vi "GV-SetSamplesDots.vi"(8 "error in (no error)":errorcluster, 11 "Gviewer in":refnum<class "Gviewer.lvclass">) -> (0 "error out":errorcluster, 3 "Gviewer out":refnum<class "Gviewer.lvclass">)   [LabVIEW 2020, in "Sgraph_lib_V1.lvlib" / "Gviewer.lvclass"]
doc: "Andre Koelewijn, 30 jun 2021\n\nDetermine if the graph dots has to be shown"
uses:
  Gviewer.lvclass
  Gviewer.lvclass/Gviewer.ctl
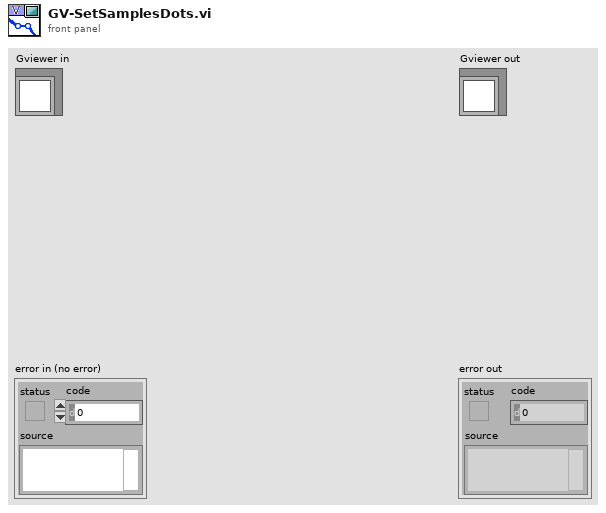
[diagram p1: front panel]
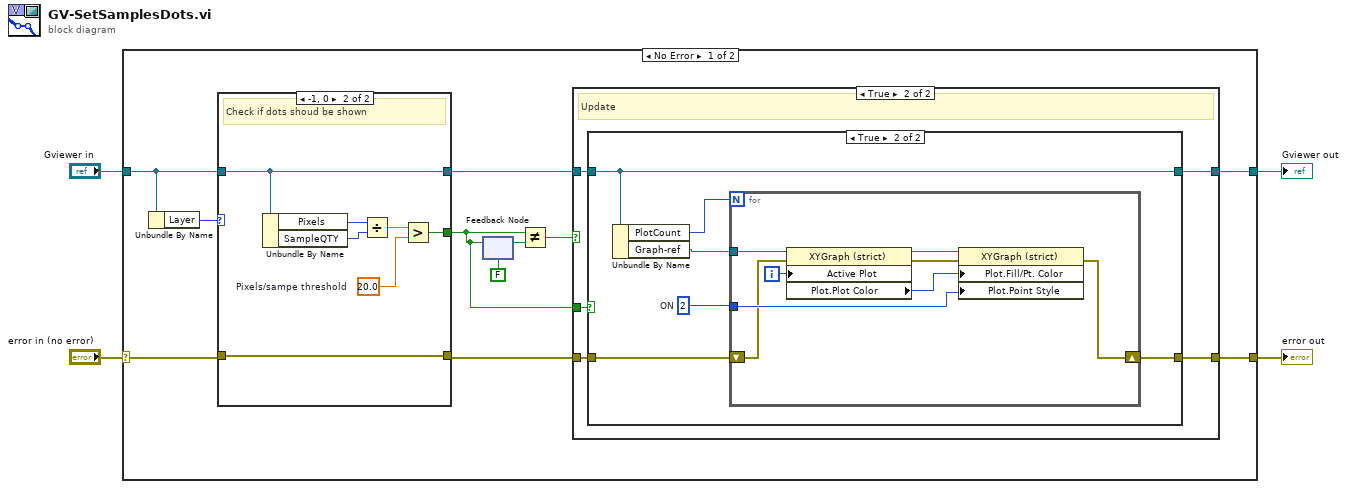
[diagram p0: block diagram]
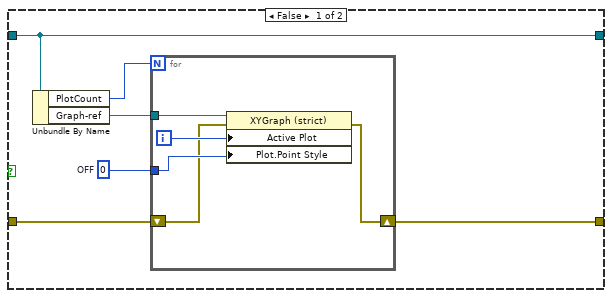
[diagram p3: hidden frame]
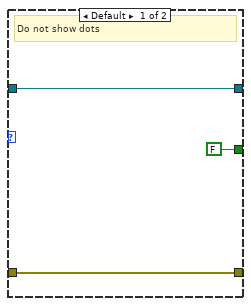
[diagram p4: hidden frame]
diagram:
  n1 = case shown="No Error" "error in (no error)" {
    selector: "error in (no error)" -> [w14 w59]
    tunnel: [w7 w59] -> w3
    tunnel: [w8 w58] -> w1
    tunnel: "Gviewer in" -> [w5 w58]
    frame No Error {
      n2 = Unbundle By Name(w5) -> ("Layer"=w15:i32)
      n3 = case shown="-1, 0" w15 {
        tunnel: w14 -> [w49 w57]
        tunnel: w5 -> [w50 w56]
        tunnel: [w50 w56] -> w10
        tunnel: [w49 w57] -> w9
        tunnel: [FALSE w51] -> w6
        frame Default {
          # "Do not show dots"
        }
        frame -1, 0 {
          w52 = 20.0  # Pixels/sampe threshold
          # "Check if dots shoud be shown"
          n4 = Unbundle By Name(w56) -> ("Pixels"=w55:i32, "SampleQTY"=w54:i32)
          n5 = Divide(x=w55, y=w54) -> (x/y=w53:dbl)
          n6 = Greater?(x=w53, y=w52) -> (0:w51:bool)
        }
      }
      n7 = feedback-in #1(w6) -> ()
      n8 = feedback #1(FALSE) -> (w13:bool)
      n9 = Not Equal?(x=w6, y=w13) -> (x != y?=w11:bool)
      n10 = case shown="True" w11 {
        tunnel: w10 -> [w17 w22]
        tunnel: w9 -> [w16 w21]
        tunnel: [w17 w18] -> w8
        tunnel: [w16 w20] -> w7
        tunnel: w6 -> [_ w19]
        frame False {
          # "do not update"
        }
        frame True {
          # "Update"
          n11 = case shown="True" w19 {
            tunnel: w22 -> [w23 w36]
            tunnel: w21 -> [w26 w35]
            tunnel: [w25 w34] -> w20
            tunnel: [w23 w36] -> w18
            frame False {
              w24 = u8 0  # OFF
              n12 = Unbundle By Name(w23) -> ("PlotCount"=w27:i32, "Graph-ref"=w28:refnum<vi>)
              n13 = for {
                N: w27 -> [_]
                tunnel: w28 -> [w33]
                tunnel: w24 -> [w31]
                shift-right: [w29] -> w25
                shift-left: w26 -> [w30]
                i -> [w32]
                n14 = property class="XYGraph (strict)"(reference=w33, error in=w30, "Active Plot"=w32, "Plot.Point Style"=w31) -> (error out=w29:errorcluster)  [unwired: 1 out]
              }
            }
            frame True {
              w37 = u8 2  # ON
              n15 = Unbundle By Name(w36) -> ("PlotCount"=w38:i32, "Graph-ref"=w39:refnum<vi>)
              n16 = for {
                N: w38 -> [_]
                tunnel: w39 -> [w44]
                tunnel: w37 -> [w47]
                shift-right: [w46] -> w34
                shift-left: w35 -> [w42]
                i -> [w43]
                n17 = property class="XYGraph (strict)"(reference=w44, error in=w42, "Active Plot"=w43) -> (reference out=w45:refnum<vi>, error out=w40:errorcluster, "Plot.Plot Color"=w41:u32)
                n18 = property class="XYGraph (strict)"(reference=w45, error in=w40, "Plot.Fill/Pt. Color"=w41, "Plot.Point Style"=w47) -> (error out=w46:errorcluster)  [unwired: 1 out]
              }
            }
          }
        }
      }
    }
    frame Error {
    }
  }
  "error out" <- w3
  "Gviewer out" <- w1
